vi "sig rtos.vi"() -> ()   [LabVIEW 2020]
uses:
  <vilib>/Analysis/Matrix/Datatypes/RealMatrix.ctl
  <vilib>/Analysis/Matrix/Numeric/Conversions/Array To Matrix - RA.vi
  <vilib>/Analysis/Matrix/NI_Matrix.lvlib
panel:
  out "overall time":u32
  out "product":T1
  in  "vector size":i32=20
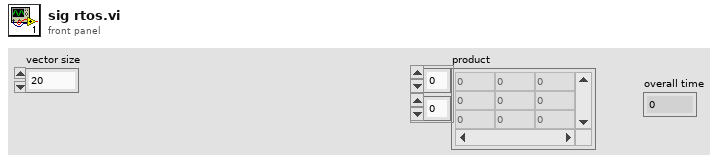
[diagram p1: front panel]
types:
  T1 = typedef "NI_Matrix.lvlib/RealMatrix.ctl" = dbl[][]
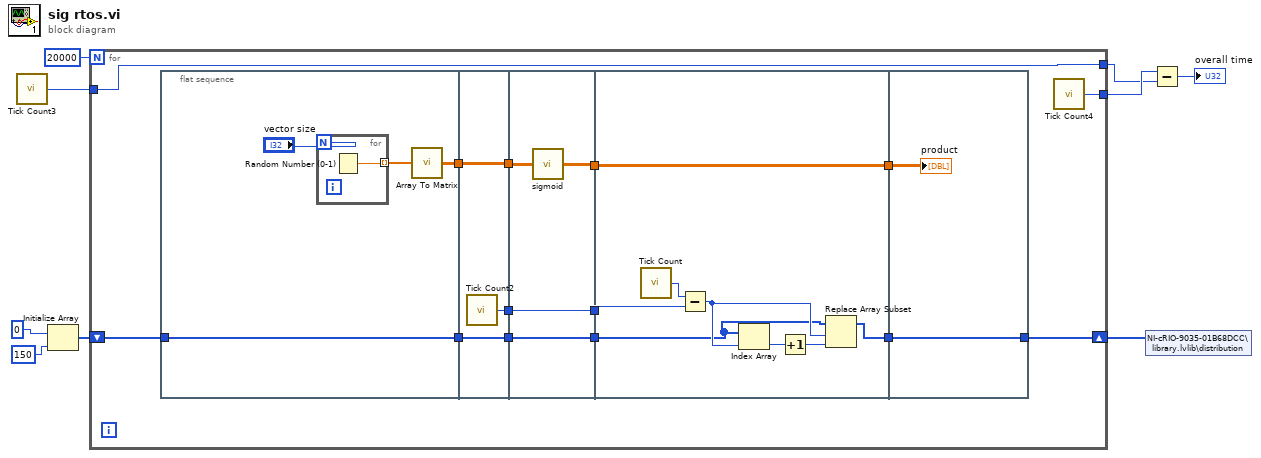
[diagram p0: block diagram]
diagram:
  n1 = call "Tick Count3"() -> ("Tick Count(uSec)"=w5:u32)
  n2 = Initialize Array(0, 150) -> (w6:i32[])
  n3 = for {
    N: 20000 -> [_]
    shift-right: [w12] -> w1
    shift-left: w6 -> [w14]
    tunnel: [w11] -> w3
    tunnel: w5 -> [w11]
    tunnel: [w10] -> w4
    n4 = flat-sequence {
      tunnel: [w26] -> w23
      tunnel: [w24] -> w15
      tunnel: w14 -> [w24]
      tunnel: w23 -> [w31]
      tunnel: [w31] -> w22
      tunnel: [w30] -> w21
      tunnel: [w29] -> w16
      tunnel: w15 -> [w29]
      tunnel: w22 -> [w32]
      tunnel: w21 -> [w35]
      tunnel: [w35] -> w20
      tunnel: [w33] -> w19
      tunnel: [w34] -> w17
      tunnel: w16 -> [w34]
      tunnel: w19 -> [w41]
      tunnel: w20 -> [w42]
      tunnel: [w41] -> w18
      tunnel: w17 -> [w37]
      tunnel: [w36] -> w13
      tunnel: w18 -> [w45]
      tunnel: w13 -> [w44]
      tunnel: [w44] -> w12
      frame #0 {
        n5 = for {
          N: "vector size" -> [_]
          tunnel: [w28] -> w27 mode=indexing
          n6 = Random Number (0-1)() -> (number: 0 to 1=w28:dbl)
        }
        n7 = call-poly <vilib>:"Array To Matrix.vi"("Real 1D Array"=w27) -> ("Real Matrix (Column Vector)"=w26:T1)
      }
      frame #1 {
        n8 = call "Tick Count2"() -> ("Tick Count(uSec)"=w30:u32)
      }
      frame #2 {
        n9 = call <vilib>:"sigmoid.vi"("x"=w32) -> ("y"=w33:T1)
      }
      frame #3 {
        n10 = call "Tick Count"() -> ("Tick Count(uSec)"=w43:u32)
        n11 = Subtract(x=w43, y=w42) -> (x-y=w38:u32)
        n12 = Index Array(array=w37, index=w38) -> (element=w39:i32)
        n13 = Increment(x=w39) -> (x+1=w40:i32)
        n14 = Replace Array Subset(array=w37, new element=w40, index=w38) -> (w36:i32[])
      }
      frame #4 {
        "product" <- w45
      }
    }
    n15 = call "Tick Count4"() -> ("Tick Count(uSec)"=w10:u32)
  }
  n16 = shared-variable "NI-cRIO-9035-01B68DCC\\library.lvlib\\distribution"(w1) -> ()  [unwired: 1 in, 1 out]
  n17 = Subtract(x=w4, y=w3) -> (x-y=→"overall time":u32)
